vi "sub vi - AI USB4704 (3)  Create Task v4.vi"(0 "Test":bool=TRUE, 9 "Rate Hz":dbl, 11 "Samples":dbl) -> (1 "physical channels 0":string="DemoDevice,BID#0/ai0:1" caption="property value", 2 "physical channels 1":string="DemoDevice,BID#0/ai0:1" caption="property value", 3 "physical channels 2":string="DemoDevice,BID#0/ai0:1" caption="property value", 4 "TASK USB 0":i32, 6 "TASK USB 1":i32, 8 "TASK USB 2":i32, 14 "AI Task Er":bool, 15 "error array":errorcluster[](array[cluster]))   [LabVIEW 2017]
uses:
  <userlib>/DAQNavi Polymorphic VI/create/DAQNavi Create Channel(AI-Voltage).vi
  <userlib>/DAQNavi Polymorphic VI/configure/timing/DAQNavi Timing(Convert Clock).vi
  <userlib>/DAQNavi Polymorphic VI/configure/DAQNavi Get Property/AI/DAQNaviGet_AI_ConvertClock_Rate.vi
panel:
  in  "Tab Control":enum32{"Tasks In", "USB #0", "USB #1", "USB #2"}(tab)
  out "value range 0":string="+/- 5 V" caption="property value"
  out "convert rate 0":dbl
  out "value range  1":string="+/- 5 V" caption="property value"
  out "convert rate 1":dbl
  out "value range  2":string="+/- 5 V" caption="property value"
  out "convert rate 2":dbl
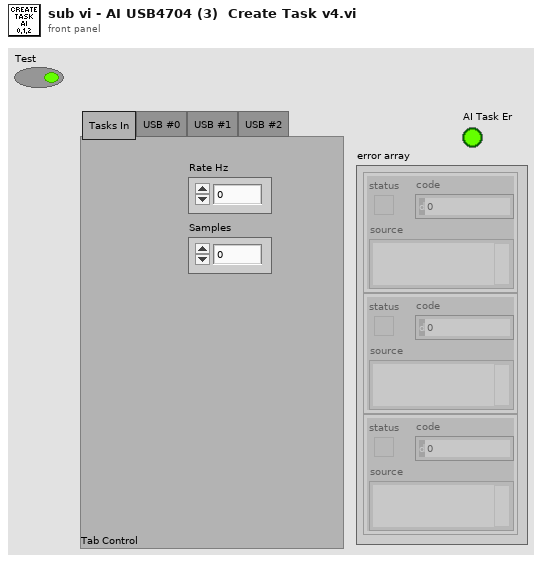
[diagram p1: front panel]
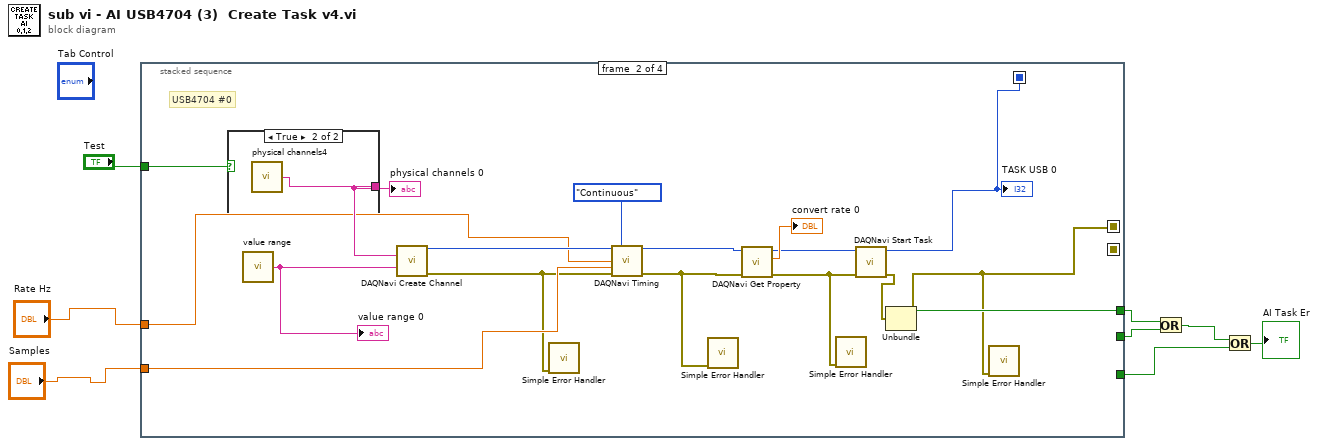
[diagram p0: block diagram]
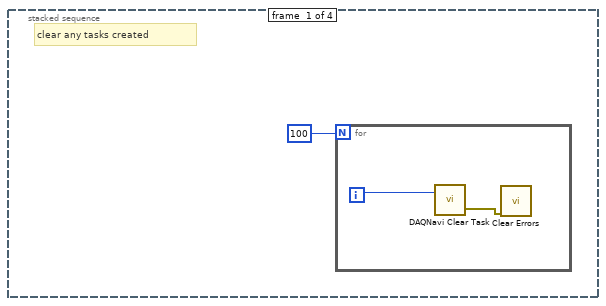
[diagram p2: hidden frame]
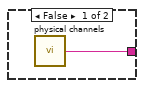
[diagram p3: hidden frame]
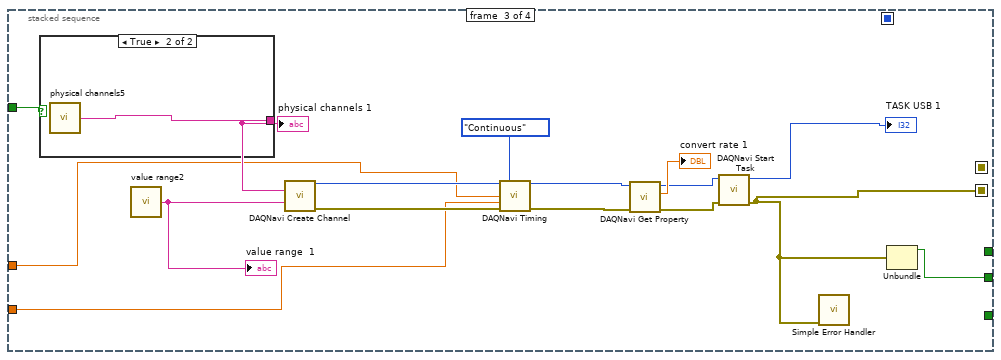
[diagram p4: hidden frame]
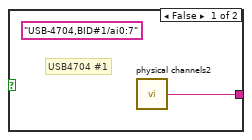
[diagram p5: hidden frame]
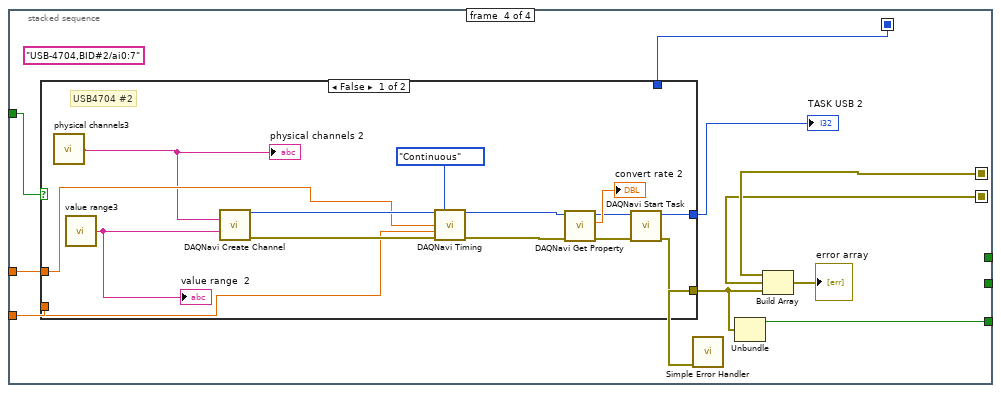
[diagram p6: hidden frame]
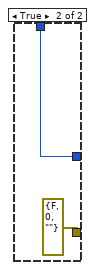
[diagram p7: hidden frame]
diagram:
  n1 = stacked-sequence {
    seq-local: [_ w17 _ _] -> [_ _ _ w57]
    seq-local: [_ _ w31 _] -> [_ _ _ w56]
    seq-local: [_ w12 _ _] -> [_ _ _ w49]
    tunnel: "Rate Hz" -> [_ w21 w37 w54]
    tunnel: "Samples" -> [_ w20 w36 w53]
    tunnel: [_ _ _ w52] -> w6
    tunnel: [_ w19 _ _] -> w5
    tunnel: [_ _ w35 _] -> w4
    tunnel: "Test" -> [_ w13 w30 w48]
    frame #0 {
      # "clear any tasks created"
      n2 = for {
        N: 100 -> [_]
        i -> [w11]
        n3 = call <userlib>:"DAQNavi Clear Task.vi"("task in"=w11) -> ("error out"=w10:errorcluster)  [unwired: 2 in]
        n4 = call <vilib>:"Clear Errors.vi"("error in (no error)"=w10) -> ()  [unwired: 5 in, 2 out]
      }
    }
    frame #1 {
      # "USB4704 #0"
      n5 = case shown="True" w13 {
        tunnel: [w28 w29] -> w26
        frame False {
          n6 = call "physical channels"() -> ("property value"=w28:string)  [unwired: 1 out]
        }
        frame True {
          n7 = call "physical channels4"() -> ("property value"=w29:string)  [unwired: 1 out]
        }
      }
      "physical channels 0" <- w26
      n8 = call "value range"() -> ("property value"=w27:string)  [unwired: 1 out]
      "value range 0" <- w27
      n9 = call-poly <userlib>:"DAQNavi Create Channel.vi"("physical channels"=w26, "value range"=w27) -> ("task out"=w22:i32, "error out"=w16:errorcluster)  [unwired: 3 in, 9 out]
      n10 = call <vilib>:"Simple Error Handler.vi"("error in (no error)"=w16) -> ()  [unwired: 4 in, 5 out]
      n11 = call-poly <userlib>:"DAQNavi Timing.vi"("task in"=w22, "sample mode"=enum16{"Finite", "Continuous"}."Continuous", "rate"=w21, "samples per channel"=w20, "error in (no error)"=w16) -> ("task out"=w24:i32, "error out"=w15:errorcluster)  [unwired: 1 in, 8 out]
      n12 = call <vilib>:"Simple Error Handler.vi"("error in (no error)"=w15) -> ()  [unwired: 4 in, 5 out]
      n13 = call-poly <userlib>:"DAQNavi Get Property.vi"("error in (no error)"=w15, "task in"=w24) -> ("error out"=w14:errorcluster, "rate"=→"convert rate 0":dbl, "task out"=w18:i32)  [unwired: 7 out]
      n14 = call <vilib>:"Simple Error Handler.vi"("error in (no error)"=w14) -> ()  [unwired: 4 in, 5 out]
      n15 = call <userlib>:"DAQNavi Start Task.vi"("error in (no error)"=w14, "task in"=w18) -> ("error out"=w17:errorcluster, "task out"=w12:i32)  [unwired: 8 in]
      "TASK USB 0" <- w12
      n16 = Unbundle(w17) -> ("status"=w19:bool)  [unwired: 2 out]
      n17 = call <vilib>:"Simple Error Handler.vi"("error in (no error)"=w17) -> ()  [unwired: 4 in, 5 out]
    }
    frame #2 {
      n18 = case shown="True" w30 {
        tunnel: [w46 w47] -> w44
        frame False {
          (unwired) "USB-4704,BID#1/ai0:7" ("property value")
          # "USB4704 #1"
          n19 = call "physical channels2"() -> ("property value"=w46:string)  [unwired: 1 out]
        }
        frame True {
          n20 = call "physical channels5"() -> ("property value"=w47:string)  [unwired: 1 out]
        }
      }
      "physical channels 1" <- w44
      n21 = call "value range2"() -> ("property value"=w45:string)  [unwired: 1 out]
      "value range  1" <- w45
      n22 = call-poly <userlib>:"DAQNavi Create Channel.vi"("physical channels"=w44, "value range"=w45) -> ("task out"=w38:i32, "error out"=w39:errorcluster)  [unwired: 3 in, 9 out]
      n23 = call-poly <userlib>:"DAQNavi Timing.vi"("task in"=w38, "sample mode"=enum16{"Finite", "Continuous"}."Continuous", "rate"=w37, "samples per channel"=w36, "error in (no error)"=w39) -> ("task out"=w41:i32, "error out"=w42:errorcluster)  [unwired: 1 in, 8 out]
      n24 = call-poly <userlib>:"DAQNavi Get Property.vi"("error in (no error)"=w42, "task in"=w41) -> ("error out"=w34:errorcluster, "rate"=→"convert rate 1":dbl, "task out"=w33:i32)  [unwired: 7 out]
      n25 = call <userlib>:"DAQNavi Start Task.vi"("error in (no error)"=w34, "task in"=w33) -> ("error out"=w31:errorcluster, "task out"=→"TASK USB 1":i32)  [unwired: 8 in]
      n26 = call <vilib>:"Simple Error Handler.vi"("error in (no error)"=w31) -> ()  [unwired: 4 in, 5 out]
      n27 = Unbundle(w31) -> ("status"=w35:bool)  [unwired: 2 out]
    }
    frame #3 {
      (unwired) "USB-4704,BID#2/ai0:7" ("property value")
      n28 = case shown="False" w48 {
        tunnel: w54 -> [w64 _]
        tunnel: w53 -> [w63 _]
        tunnel: [w60 w72] -> w51
        tunnel: [w59 errorcluster {"status"=FALSE, "code"=0, "source"=""} ("error out")] -> w50
        tunnel: w49 -> [_ w72]
        frame False {
          # "USB4704 #2"
          n29 = call "physical channels3"() -> ("property value"=w58:string)  [unwired: 1 out]
          "physical channels 2" <- w58
          n30 = call "value range3"() -> ("property value"=w71:string)  [unwired: 1 out]
          "value range  2" <- w71
          n31 = call-poly <userlib>:"DAQNavi Create Channel.vi"("physical channels"=w58, "value range"=w71) -> ("task out"=w65:i32, "error out"=w66:errorcluster)  [unwired: 3 in, 9 out]
          n32 = call-poly <userlib>:"DAQNavi Timing.vi"("task in"=w65, "sample mode"=enum16{"Finite", "Continuous"}."Continuous", "rate"=w64, "samples per channel"=w63, "error in (no error)"=w66) -> ("task out"=w68:i32, "error out"=w69:errorcluster)  [unwired: 1 in, 8 out]
          n33 = call-poly <userlib>:"DAQNavi Get Property.vi"("error in (no error)"=w69, "task in"=w68) -> ("error out"=w61:errorcluster, "rate"=→"convert rate 2":dbl, "task out"=w62:i32)  [unwired: 7 out]
          n34 = call <userlib>:"DAQNavi Start Task.vi"("error in (no error)"=w61, "task in"=w62) -> ("error out"=w59:errorcluster, "task out"=w60:i32)  [unwired: 8 in]
        }
        frame True {
        }
      }
      "TASK USB 2" <- w51
      n35 = call <vilib>:"Simple Error Handler.vi"("error in (no error)"=w50) -> ()  [unwired: 4 in, 5 out]
      n36 = Unbundle(w50) -> ("status"=w52:bool)  [unwired: 2 out]
      n37 = Build Array(w57, w56, w50) -> (→"error array":errorcluster[])
    }
  }
  n38 = Or(x=w5, y=w4) -> (x .or. y?=w7:bool)
  n39 = Or(x=w7, y=w6) -> (x .or. y?=→"AI Task Er":bool)
